vi "(TestVI)Accelerometer Test 2.vi"() -> ()   [LabVIEW 2020]
uses:
  SubVIs/Serial/Controls/(Ctrl)Serial_FGV Function.ctl
  <vilib>/Instr/_visa.llb/VISA Find Search Mode.ctl
  f00dcade-cb96-452d-bd30-e8a228c9f858.vi
panel:
  in  "Sensor Offset Calibration":bool
  in  "Stop":bool
  out "웨이브폼 차트":dbl[][](graph)
  out "Mode":u8
  in  "Continuous":bool
  in  "Recording Time":u16=100
  in  "Sensor Scale Setting":bool
  in  "Auto Trigger":bool
  in  "정지":bool
  in  "Sensor Activation":bool
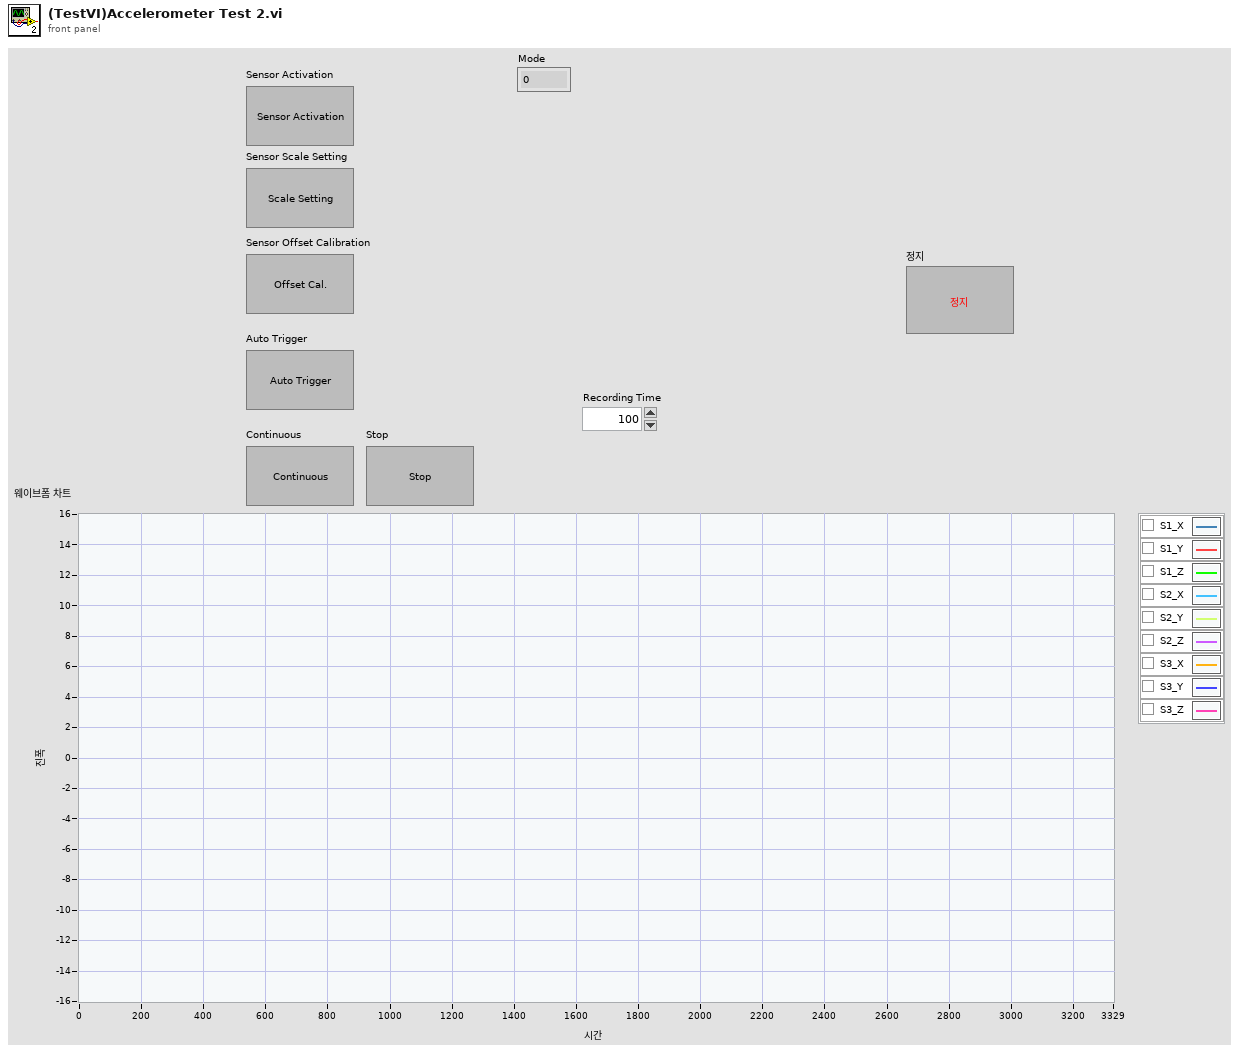
[diagram p1: front panel]
types:
  T1 = typedef "VISA Find Search Mode.ctl" = u32
  T2 = typedef "(Ctrl)Serial_FGV Function.ctl" = enum16{"Initialize", "Read", "Read All", "Write", "Flush Buffer", "Get Ref.", "Close"}
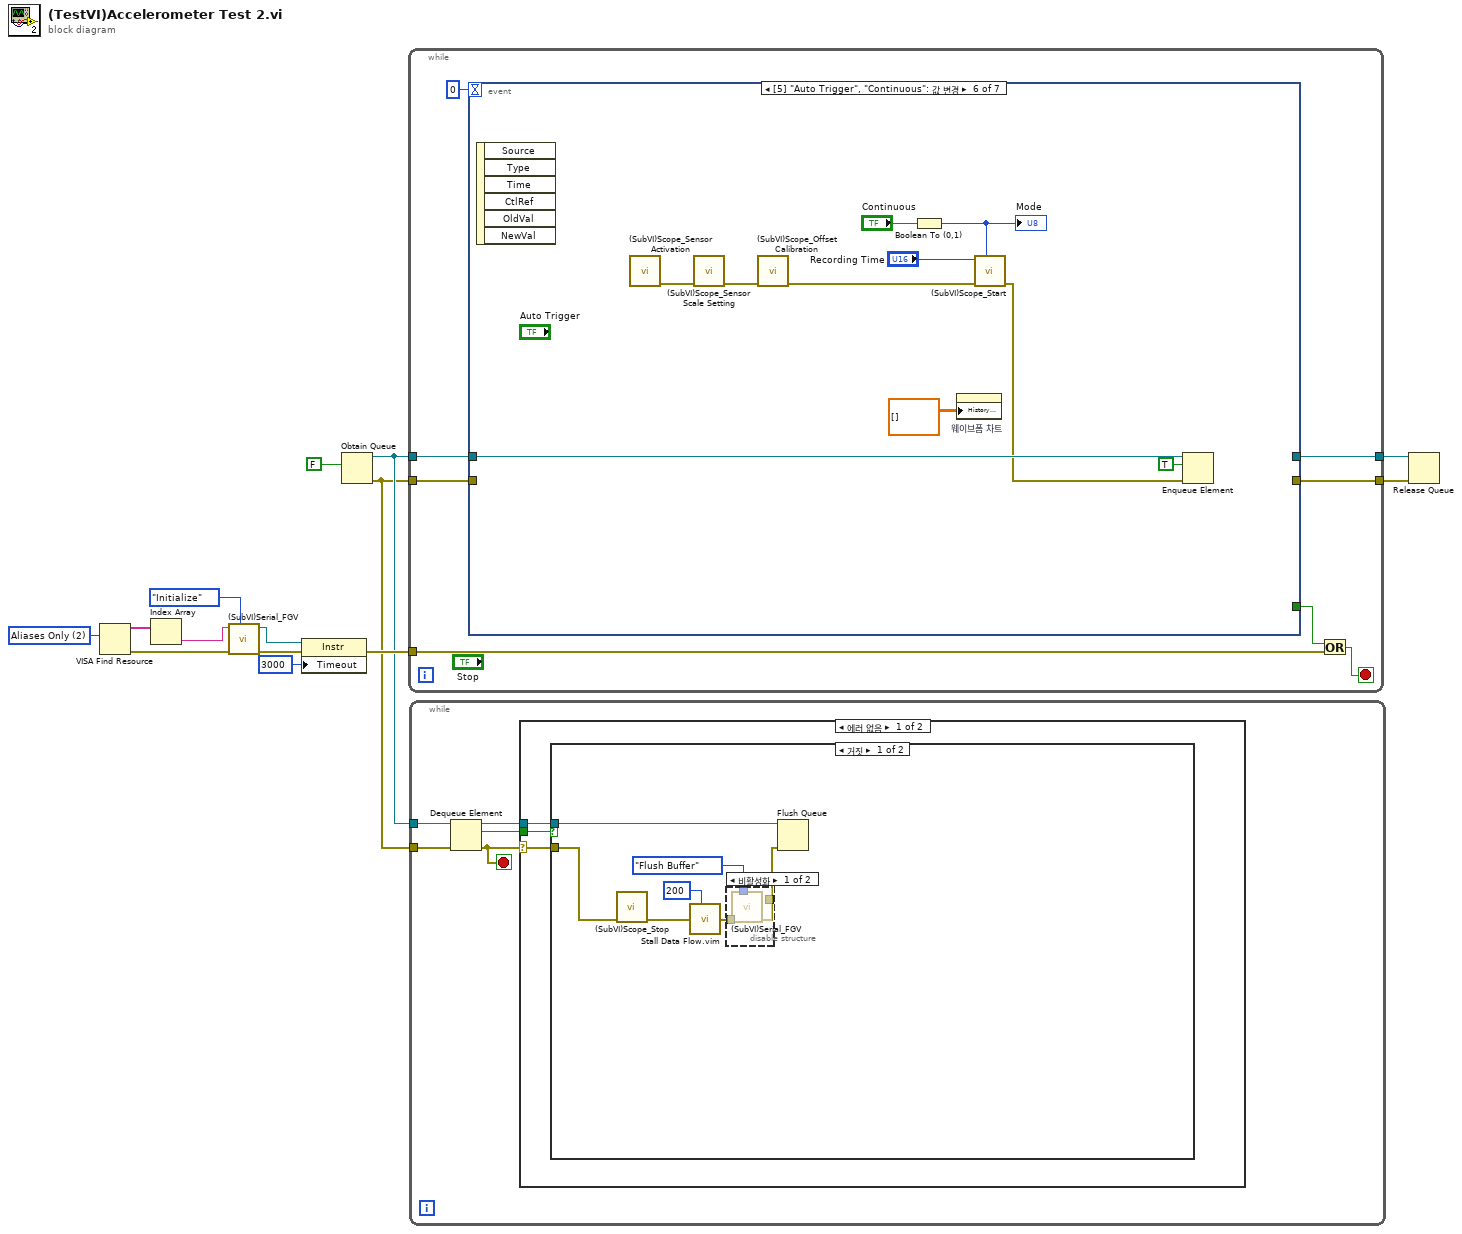
[diagram p0: block diagram]
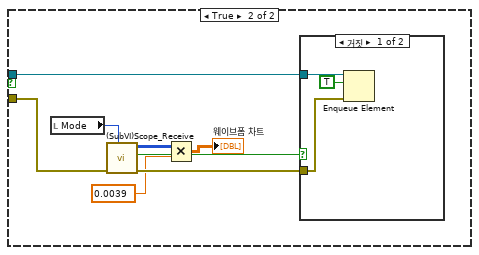
[diagram p3: hidden frame]
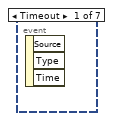
[diagram p6: hidden frame]
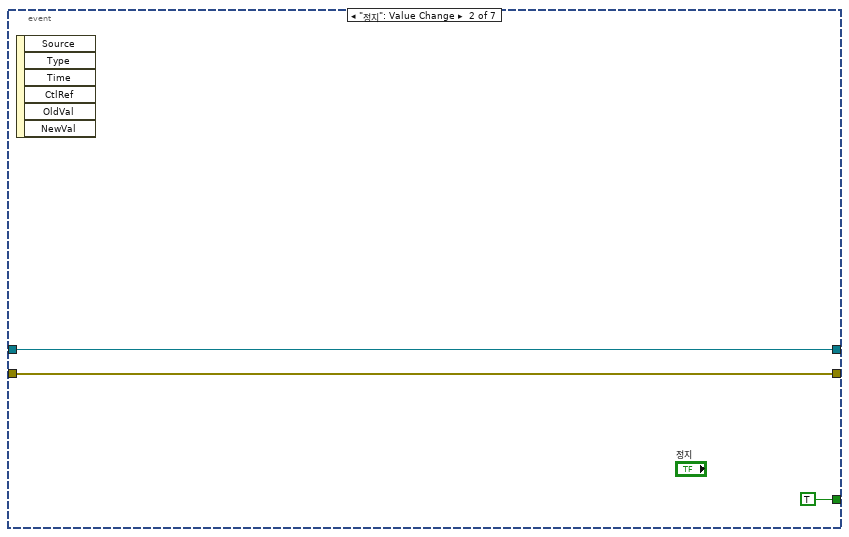
[diagram p7: hidden frame]
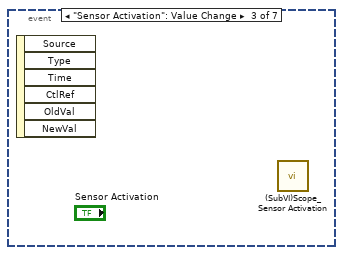
[diagram p8: hidden frame]
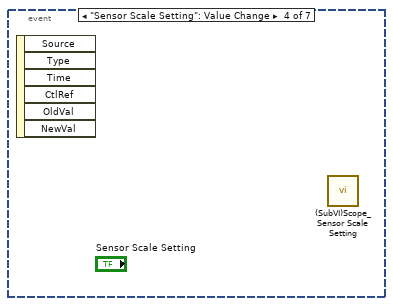
[diagram p9: hidden frame]
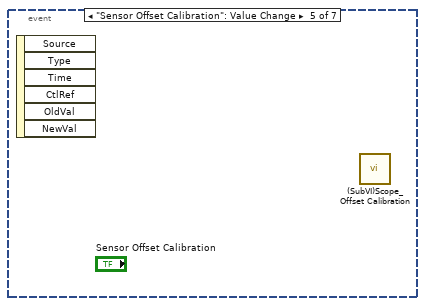
[diagram p10: hidden frame]
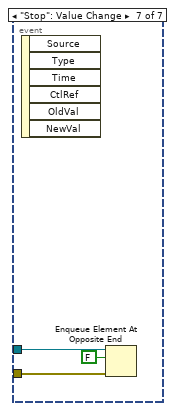
[diagram p11: hidden frame]
diagram:
  w13 = T1 2 items=["Canonical Names Only"=0, "Aliases Only"=2, "Include Matching Aliases"=3, "Include All Aliases"=4] ("Search Mode")
  n1 = VISA Find Resource(10:w13) -> (0:w12:errorcluster, 3:w11:string[])  [unwired: 2 in, 1 out]
  n2 = Index Array(array=w11) -> (element=w10:string)  [unwired: 1 in]
  n3 = call "(SubVI)Serial_FGV.vi"("Function"=(Ctrl)Serial_FGV_Function."Initialize", "error in (no error)"=w12, "VISA resource name"=w10) -> ("error out"=w9:errorcluster, "VISA resource name out"=w7:refnum<visa-resource-name>)  [unwired: 6 in, 1 out]
  n4 = property class="Instr"(reference=w7, error in=w9, "Timeout"=u32 3000 ("General Settings:Timeout Value")) -> (error out=w8:errorcluster)  [unwired: 1 out]
  n5 = Obtain Queue(element data type=FALSE) -> (queue out=w4:refnum<queue>, error out=w3:errorcluster)  [unwired: 4 in, 1 out]
  n6 = while {
    tunnel: w8 -> [w21]
    tunnel: w4 -> [w18]
    tunnel: w3 -> [w17]
    tunnel: [w16] -> w2
    tunnel: [w15] -> w1
    stop <- w20 stop-if-true
    n7 = event shown="[5] \"Auto Trigger\", \"Continuous\": 값 변경" {
      selector: _ -> [_ _ _ _ _ _ _]
      dyn-events: _ -> [_ _ _ _ _ _ _]
      timeout: 0 -> [_ _ _ _ _ _ _]
      tunnel: [_ TRUE _ _ _ _ _] -> w19
      tunnel: w18 -> [_ w24 _ _ _ w35 w38]
      tunnel: w17 -> [_ w23 _ _ _ _ w37]
      tunnel: [_ w24 _ _ _ _ _] -> w16
      tunnel: [_ w23 _ _ _ _ _] -> w15
      event Timeout {
        n8 = event-data() -> ()  [unwired: 1 in, 3 out]
      }
      event "정지": Value Change {
        n9 = event-data() -> ()  [unwired: 1 in, 6 out]
      }
      event "Sensor Activation": Value Change {
        n10 = event-data() -> ()  [unwired: 1 in, 6 out]
        n11 = call "(SubVI)Scope_Sensor Activation.vi"() -> ()  [unwired: 10 in, 2 out]
      }
      event "Sensor Scale Setting": Value Change {
        n12 = event-data() -> ()  [unwired: 1 in, 6 out]
        n13 = call "(SubVI)Scope_Sensor Scale Setting.vi"() -> ()  [unwired: 10 in, 1 out]
      }
      event "Sensor Offset Calibration": Value Change {
        n14 = event-data() -> ()  [unwired: 1 in, 6 out]
        n15 = call "(SubVI)Scope_Offset Calibration.vi"() -> ()  [unwired: 11 in, 1 out]
      }
      event "Auto Trigger", "Continuous": Value Change {
        n16 = event-data() -> ()  [unwired: 1 in, 6 out]
        n17 = call "(SubVI)Scope_Sensor Activation.vi"() -> ("error out"=w27:errorcluster)  [unwired: 10 in, 1 out]
        n18 = call "(SubVI)Scope_Sensor Scale Setting.vi"("error in (no error)"=w27) -> ("error out"=w26:errorcluster)  [unwired: 9 in]
        n19 = call "(SubVI)Scope_Offset Calibration.vi"("error in (no error)"=w26) -> ("error out"=w30:errorcluster)  [unwired: 10 in]
        n20 = Boolean To (0,1)(Boolean="Continuous") -> (0, 1=w32:i16)
        "Mode" <- w32
        n21 = property on="웨이브폼 차트" class="WFChart (엄격한)"("History Data"=dbl[][] [] ("히스토리 데이터")) -> ()  [unwired: 2 in, 2 out]
        n22 = call "(SubVI)Scope_Start.vi"("Mode"=w32, "error in (no error)"=w30, "Recording Time"="Recording Time") -> ("error out"=w29:errorcluster)  [unwired: 8 in]
        n23 = Enqueue Element(queue=w35, element=TRUE ("원소"), error in (no error)=w29) -> ()  [unwired: 1 in, 3 out]
      }
      event "Stop": Value Change {
        n24 = event-data() -> ()  [unwired: 1 in, 6 out]
        n25 = Enqueue Element At Opposite End(queue=w38, element=FALSE ("원소"), error in (no error)=w37) -> ()  [unwired: 1 in, 3 out]
      }
    }
    n26 = Or(x=w19, y=w21) -> (x .or. y?=w20:bool)
  }
  n27 = while {
    tunnel: w4 -> [w43]
    tunnel: w3 -> [w42]
    stop <- w41 stop-if-true
    n28 = Dequeue Element(queue=w43, error in (no error)=w42) -> (queue out=w39:refnum<queue>, element=w40:bool, error out=w41:errorcluster)  [unwired: 1 in, 1 out]
    n29 = case shown="에러 없음" w41 {
      selector: w41 -> [w45 _]
      tunnel: w40 -> [w46 _]
      tunnel: w39 -> [w44 _]
      frame No Error {
        n30 = case shown="거짓" w46 {
          tunnel: w45 -> [w53 w64]
          tunnel: w44 -> [w52 w60]
          frame False {
            n31 = call "(SubVI)Scope_Stop.vi"("error in (no error)"=w53) -> ("error out"=w51:errorcluster)  [unwired: 10 in]
            n32 = call "Stall Data Flow.vim"("value in"=w51, "milliseconds to wait"=u32 200) -> ("value out"=w48:errorcluster)  [unwired: 1 out]
            n33 = disable-structure shown="비활성화" {
              disable-tunnel: [w56 _] -> w50
              disable-tunnel: (Ctrl)Serial_FGV_Function."Flush Buffer" ("Function") -> [w55 _]
              disable-tunnel: w48 -> [w54 _]
              frame Disabled {
                n34 = call "(SubVI)Serial_FGV.vi"("Function"=w55, "error in (no error)"=w54) -> ("error out"=w56:errorcluster)  [unwired: 7 in, 2 out]
              }
              frame Enabled {
              }
            }
            n35 = Flush Queue(queue=w52, error in (no error)=w50) -> ()  [unwired: 3 out]
          }
          frame True {
            n36 = local read "Mode"() -> (w63:u8)
            n37 = call "(SubVI)Scope_Receive.vi"("User Code"=w63, "error in (no error)"=w64) -> ("error out"=w62:errorcluster, "End"=w61:bool, "Data"=w58:i16[][])  [unwired: 7 in]
            n38 = Multiply(x=w58, y=0.0039) -> (x*y=→"웨이브폼 차트":dbl[][])
            n39 = case shown="거짓" w61 {
              tunnel: w62 -> [w66 _]
              tunnel: w60 -> [w67 _]
              frame False {
                n40 = Enqueue Element(queue=w67, element=TRUE ("원소"), error in (no error)=w66) -> ()  [unwired: 1 in, 3 out]
              }
              frame True {
              }
            }
          }
        }
      }
      frame Error {
      }
    }
  }
  n41 = Release Queue(queue=w2, error in (no error)=w1) -> ()  [unwired: 1 in, 3 out]
